vi "Read Enabled Controllers.vi"(8 "error in (no error)":errorcluster, 11 "Output in":refnum<class "Output.lvclass">) -> (0 "error out":errorcluster, 2 "Enabled Channels":string[](array[string]), 3 "Output out":refnum<class "Output.lvclass">)   [LabVIEW 2024, in "Output.lvclass"]
doc: "Output.lvclass:Read Enabled Channels.vi\n\nThis is the Read Enabled Channels VI for the Output class.\n\nInstrument Communication Module Version 1.0\nOctober, 2020 Original Code Consulting Davita Bird\n www.originalcode.com"
uses:
  Output.lvclass
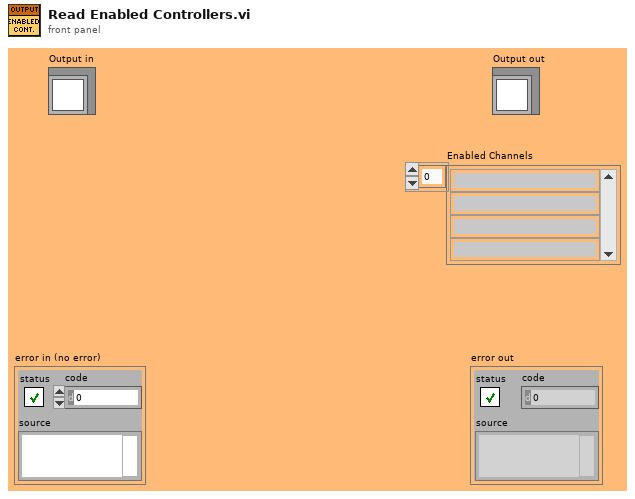
[diagram p1: front panel]
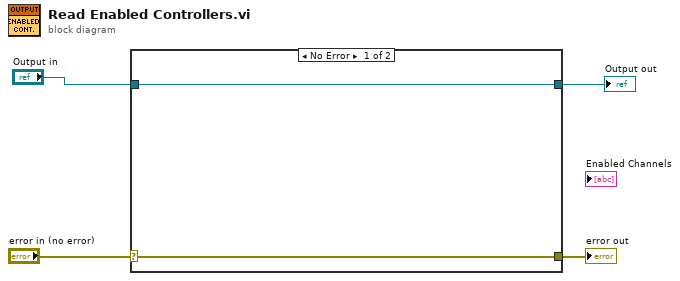
[diagram p0: block diagram]
diagram:
  n1 = case shown="No Error" "error in (no error)" {
    selector: "error in (no error)" -> [w6 w7]
    tunnel: [w6 w7] -> w3
    tunnel: [w5 w8] -> w1
    tunnel: "Output in" -> [w5 w8]
    frame No Error {
    }
    frame Error {
    }
  }
  "error out" <- w3
  "Output out" <- w1
